vi "횡단보도 알고리즘.vi"() -> ()   [LabVIEW 2016]
uses:
  <vilib>/express/express arith-compare/Formula/XNode/ExpressFormulaBlockNode.xnode
  <vilib>/vision/NI_Vision_Development_Module.lvlib
panel:
  in  "횡단보도 거리":dbl
  in  "Image Type":T1 items=["Grayscale (U8)", "Grayscale (I16)", "Grayscale (SGL)", "Complex (CSG)", "RGB (U32)", "HSL (U32)", "RGB (U64)", "Grayscale (U16)"]
  in  "Stop (F)":bool
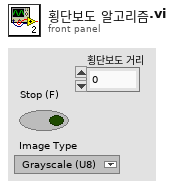
[diagram p1: front panel]
types:
  T1 = typedef "Image Type" = u32
  T2 = typedef "IMAQ Image.ctl" = refnum<image>
  T3 = cluster{"Position":cluster{"x":sgl, "y":sgl}, "Angle":sgl, "Scale":sgl, "Score":sgl, "Bounding Box":cluster{"x":sgl, "y":sgl}[]}[]
  T4 = cluster{"Position":cluster{"x":sgl, "y":sgl}, "Angle":sgl, "Scale":sgl, "Score":sgl, "Bounding Box":cluster{"x":sgl, "y":sgl}[]}
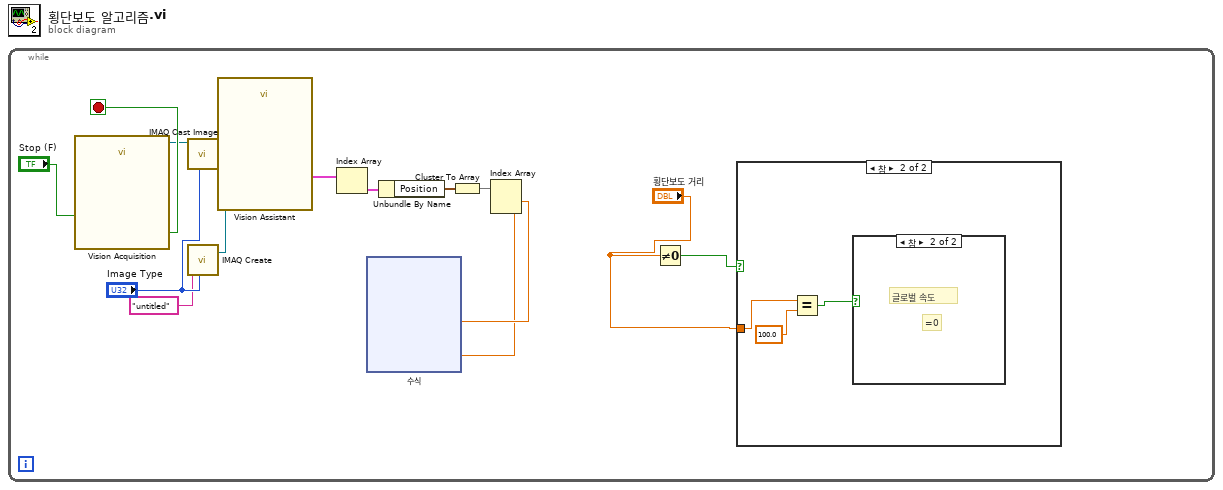
[diagram p0: block diagram]
diagram:
  n1 = while {
    stop <- w14 stop-if-true
    n2 = call "Vision Acquisition"("Stop (F)"="Stop (F)") -> ("Image Out"=w13:T2, "Stopped"=w14:bool)  [unwired: 24 in, 1 out]
    n3 = call "IMAQ Cast Image"("Image Type"="Image Type", "Image Src"=w13) -> ("Image Dst Out"=w12:T2)  [unwired: 8 in, 1 out]
    n4 = call "IMAQ Create"("Image Name"="untitled", "Image Type"="Image Type") -> ("New Image"=w11:T2)  [unwired: 3 in, 1 out]
    n5 = call "Vision Assistant"("Image In"=w12, "Image Dst"=w11) -> ("Calibrated Matches (Pattern Matching 1)"=w6:T3)  [unwired: 23 in, 2 out]
    n6 = Index Array(array=w6) -> (element=w9:T4)  [unwired: 1 in]
    n7 = Unbundle By Name(w9) -> ("Position"=w8:cluster{"x":sgl, "y":sgl})
    n8 = Cluster To Array(cluster=w8) -> (array=w7:sgl[])
    n9 = Index Array(array=w7) -> (element #1=w4:sgl, element #2=w3:sgl)  [unwired: 2 in]
    n10 = xnode "수식"("X1"=w4, "X2"=w3) -> ()  [unwired: 1 in, 2 out]
    n11 = Not Equal To 0?(x="횡단보도 거리") -> (x != 0?=w2:bool)
    n12 = case shown="참" w2 {
      tunnel: "횡단보도 거리" -> [_ w28]
      frame False {
      }
      frame True {
        n13 = Equal?(x=w28, y=sgl 100.0) -> (x = y?=w26:bool)
        n14 = case shown="참" w26 {
          frame False {
          }
          frame True {
            # "=0"
            # "글로벌 속도"
          }
        }
      }
    }
  }
